vi "Is CSM Module - EventStructure.vi"(8 "error in (no error)":errorcluster, 11 "EventStructure":refnum<vi>) -> (0 "error out":errorcluster, 2 "Is CSM Module?":bool, 3 "CSM Basic Refs":T1)   [LabVIEW 2017, in "CSM-Helper Utility.lvlib"]
doc: "#### Is CSM Module - EventStructure.vi\n\nDetermine if it is a CSM module through Event Structure reference\n\n-- <b>Controls</b> --\n- <b>EventStructure</b>: EventStructure reference\n\n-- <b>Indicators</b> --\n- <b>Is CSM Module?</b>: True If it is a CSM module\n- <b>CSM Basic Refs</b>: If This is a CSM module, It will return the basic references"
uses:
  CSM-Helper Utility.lvlib
  CSM Basic Refs.ctl
  CSM Module Type.ctl
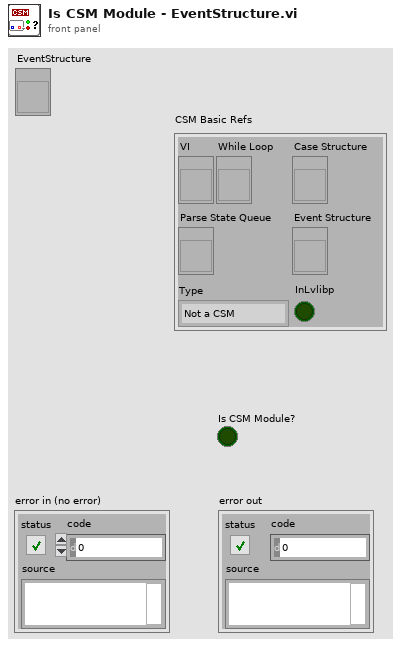
[diagram p1: front panel]
types:
  T1 = typedef "CSM-Helper Utility.lvlib/CSM Basic Refs.ctl" = cluster{"VI":refnum<vi>, "While Loop":refnum<vi>, "Case Structure":refnum<vi>, "Parse State Queue":refnum<vi>, "Event Structure":refnum<vi>, "Type":T2, "InLvlibp":bool}
  T2 = typedef "CSM-Helper Utility.lvlib/CSM Module Type.ctl" = enum16{"Not a CSM", "JKISM", "CSM"}
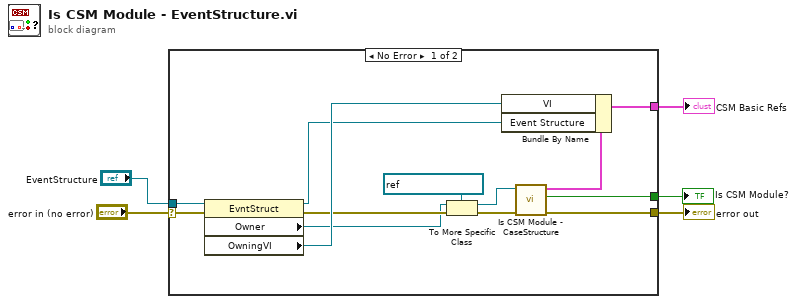
[diagram p0: block diagram]
diagram:
  n1 = case shown="No Error" "error in (no error)" {
    selector: "error in (no error)" -> [w18 w19]
    tunnel: "EventStructure" -> [w17 _]
    tunnel: [w9 w19] -> w3
    tunnel: [w8 _] -> w2
    tunnel: [w16 _] -> w1
    frame No Error {
      n2 = property on="Property Node" class="EvntStruct"(reference=w17, error in=w18) -> (reference out=w6:refnum<vi>, error out=w14:errorcluster, "Owner"=w10:refnum<vi>, "OwningVI"=w15:refnum<vi>)
      n3 = To More Specific Class(target class=refnum<vi> refnum ("CaseStructure"), reference=w10, error in=w14) -> (specific class reference=w11:refnum<vi>, error out=w13:errorcluster)
      n4 = call "Is CSM Module - CaseStructure.vi"("error in (no error)"=w13, "CaseStructure"=w11) -> ("error out"=w9:errorcluster, "Is CSM Module?"=w8:bool, "CSM Basic Refs"=w7:T1)  [unwired: 7 in]
      n5 = Bundle By Name(cluster=w7, "VI"=w15, "Event Structure"=w6) -> (w16:T1)
    }
    frame Error {
    }
  }
  "error out" <- w3
  "CSM Basic Refs" <- w1
  "Is CSM Module?" <- w2
